vi "EMC_Gearing.vi"(5 "denominator":i32=1, 6 "Gear in/out":enum16{"Gear in", "Gear out"}(ring), 7 "numerator":i32=1, 8 "error in (no error)":errorcluster, 9 "master type":T1=11599956 items=["Trajectory Master"=11599956, "Encoder Master"=11599957], 10 "master axis":refnum<k21>, 11 "axis":refnum<k21>) -> (0 "error out":errorcluster)   [LabVIEW 2015]
uses:
  EMC_Typedef_Motor_Parameters.ctl
  <vilib>/Motion/Express/_s/nimc.fb.gearing.gearingMasterType.ctl
  <vilib>/Motion/PropertyNodes/nimc.createGearingInstance.axis.vi
  <vilib>/Motion/PropertyNodes/nimc.destroyInterfaceInstance.vi
  <resource>/objmgr/nimotion.rc
panel:
  in  "table":refnum<k21>
  in  "coordinate":refnum<k21>
  in  "Motion Parameters":T2={"position"=1000.0, "velocity"=1000.0, "acceleration"=10000.0, "deceleration"=10000.0, "accel. jerk"=10000.0, "decel. jerk"=10000.0}
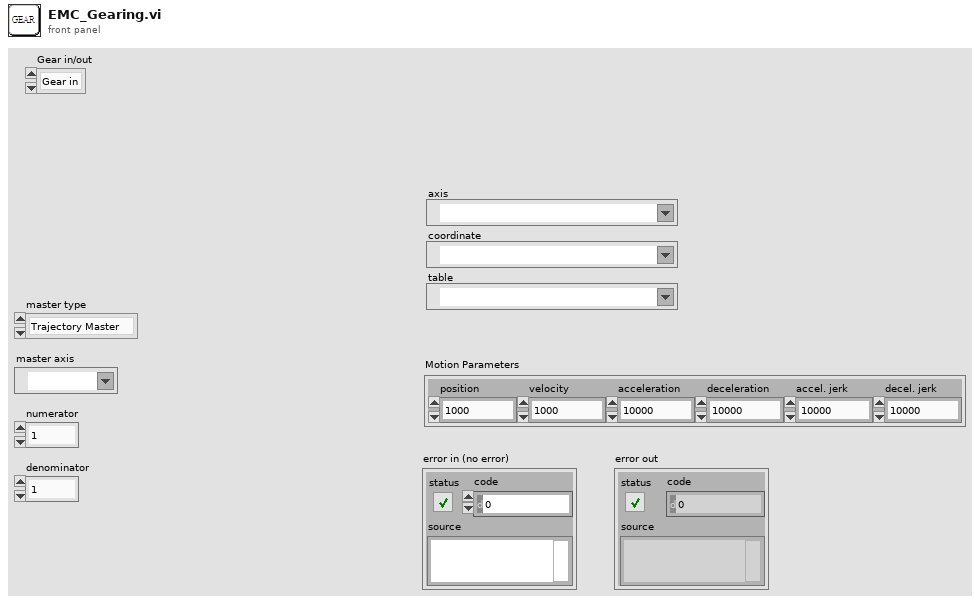
[diagram p1: front panel]
types:
  T1 = typedef "nimc.fb.gearing.gearingMasterType.ctl" = i32
  T2 = typedef "EMC_Typedef_Motor_Parameters.ctl" = cluster{"position":dbl, "velocity":dbl, "acceleration":dbl, "deceleration":dbl, "accel. jerk":dbl, "decel. jerk":dbl}
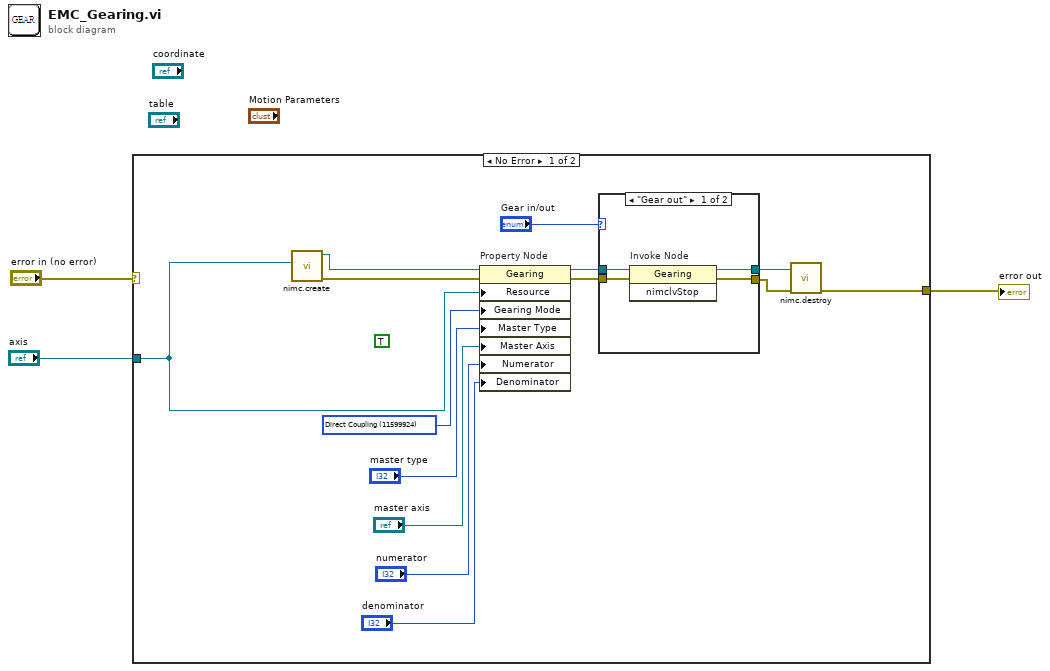
[diagram p0: block diagram]
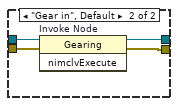
[diagram p2: hidden frame]
diagram:
  n1 = case shown="No Error" "error in (no error)" {
    selector: "error in (no error)" -> [_ w26]
    tunnel: "axis" -> [w8 _]
    tunnel: [w4 w26] -> w2
    frame No Error {
      (unwired) TRUE
      w13 = 11599924 items=["Direct Coupling"=11599924] ("gearing mode")
      n2 = call-poly <vilib>:"nimc.create.vi"("axis"=w8) -> ("error out"=w12:errorcluster, "gearing"=w11:refnum<k20>)  [unwired: 8 in, 1 out]
      n3 = property on="Property Node" class="Gearing"(reference=w11, error in=w12, "Resource"=w8, "Gearing Mode"=w13, "Master Type"="master type", "Master Axis"="master axis", "Numerator"="numerator", "Denominator"="denominator") -> (reference out=w10:refnum<k20>, error out=w9:errorcluster)
      n4 = case shown="\"Gear out\"" "Gear in/out" {
        tunnel: w10 -> [w21 w25]
        tunnel: w9 -> [w20 w24]
        tunnel: [w19 w23] -> w6
        tunnel: [w18 w22] -> w5
        frame "Gear out" {
          n5 = invoke on="Invoke Node" class="Gearing" method="nimclvStop"(reference=w21, error in=w20) -> (reference out=w19:refnum<k20>, error out=w18:errorcluster)  [unwired: 1 in, 1 out]
        }
        frame "Gear in", Default {
          n6 = invoke on="Invoke Node" class="Gearing" method="nimclvExecute"(reference=w25, error in=w24) -> (reference out=w23:refnum<k20>, error out=w22:errorcluster)  [unwired: 1 in, 1 out]
        }
      }
      n7 = call-poly <vilib>:"nimc.destroy.vi"("error in"=w5, "motion handle"=w6) -> ("error out"=w4:errorcluster)  [unwired: 9 in]
    }
    frame Error {
    }
  }
  "error out" <- w2
